vi "RegisterZeroWrite.vi"(7 "Data":T1 {"Data" max=127 format="%.0x"; "Slave Address" max=15 format="%.0x"}, 8 "error in (no error)":errorcluster, 9 "Number of Samples In":i32, 10 "Data Array":u8[][](array[numeric]), 11 "RFFE_Data In":T2 {"Toggle (high to low)" items=["0", "1", "Z", "L", "H", "X", "T", "V"]; "X Array" items=["0", "1", "Z", "L", "H", "X", "T", "V"]; "Z Array" items=["0", "1", "Z", "L", "H", "X", "T", "V"]; "L Array" items=["0", "1", "Z", "L", "H", "X", "T", "V"]; "H Array" items=["0", "1", "Z", "L", "H", "X", "T", "V"]; "One Array" items=["0", "1", "Z", "L", "H", "X", "T", "V"]; "Zero Array" items=["0", "1", "Z", "L", "H", "X", "T", "V"]}) -> (0 "error out":errorcluster, 1 "Number of Samples Out":i32, 2 "Data Array Out":u8[][](array[numeric]), 3 "RFFE_Data Out":T2 {"Toggle (high to low)" items=["0", "1", "Z", "L", "H", "X", "T", "V"]; "X Array" items=["0", "1", "Z", "L", "H", "X", "T", "V"]; "Z Array" items=["0", "1", "Z", "L", "H", "X", "T", "V"]; "L Array" items=["0", "1", "Z", "L", "H", "X", "T", "V"]; "H Array" items=["0", "1", "Z", "L", "H", "X", "T", "V"]; "One Array" items=["0", "1", "Z", "L", "H", "X", "T", "V"]; "Zero Array" items=["0", "1", "Z", "L", "H", "X", "T", "V"]})   [LabVIEW 2011]
doc: "Builds MIPI RFFE Register 0 Write with the specified data."
uses:
  Ctrls/RFFE_Data.ctl
  Ctrls/ClockDataChannels.ctl
  Ctrls/RegZeroWrite.ctl
  Ctrls/Commands.ctl
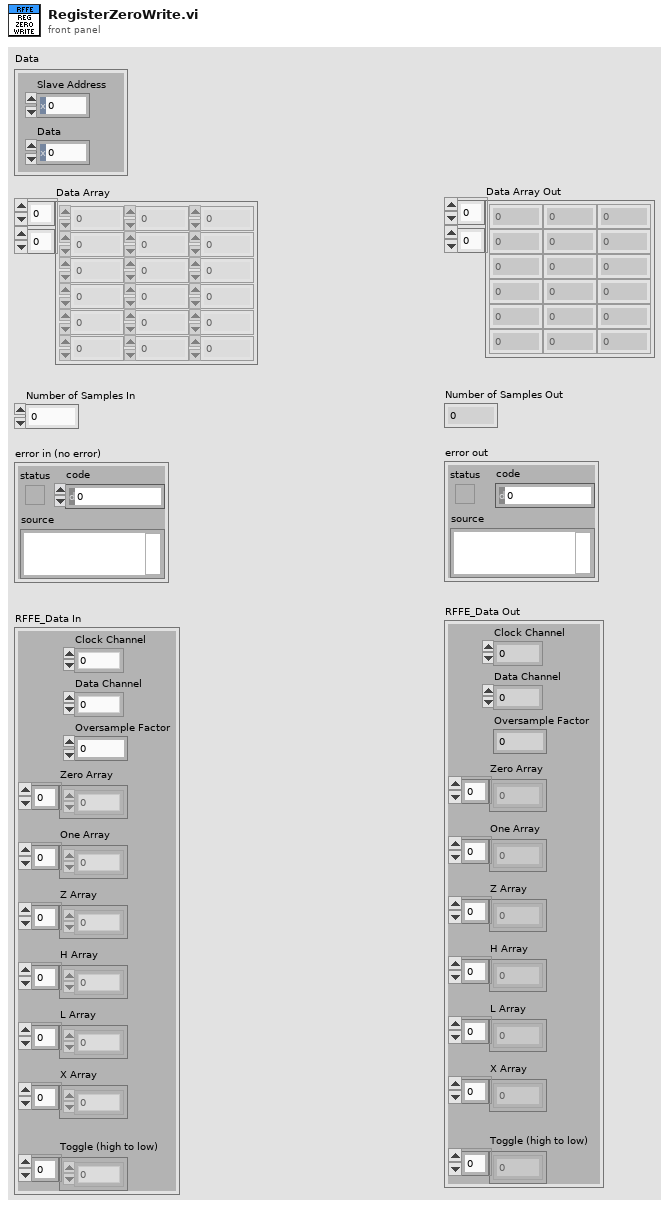
[diagram p1: front panel]
types:
  T1 = typedef "RegZeroWrite.ctl" = cluster{"Slave Address":u8, "Data":u8}
  T2 = typedef "RFFE_Data.ctl" = cluster{"Clock Channel":T3, "Data Channel":T3, "Oversample Factor":u8, "Zero Array":u8[], "One Array":u8[], "Z Array ":u8[], "H Array":u8[], "L Array":u8[], "X Array":u8[], "Toggle (high to low)":u8[]}
  T3 = typedef "ClockDataChannels.ctl" = enum16{"0", "1"}
  T4 = typedef "Commands.ctl" = cluster{"Command":enum16{"Extended Register Write", "Extended Register Read", "Extended Register Write Long", "Extended Register Read Long", "Register Write", "Register Read", "Register 0 Write"}, "Data/Address/ByteCount":u8}
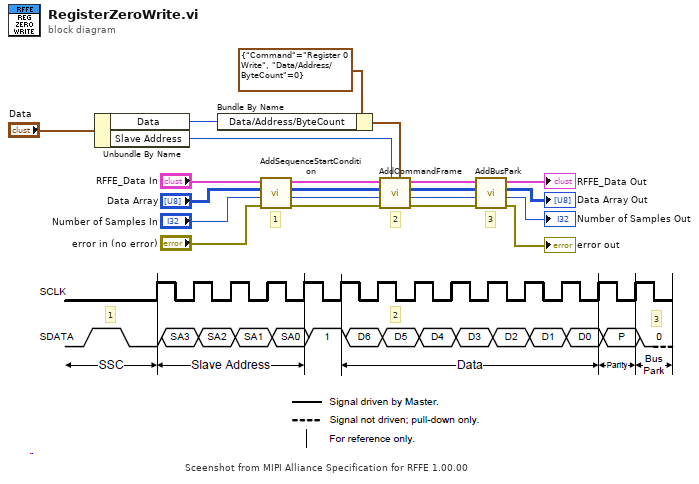
[diagram p0: block diagram]
diagram:
  # "1"
  # "3"
  # "2"
  # "Sceenshot from MIPI Alliance Specification for RFFE 1.00.00"
  # "3"
  # "2"
  # "1"
  n1 = Unbundle By Name("Data") -> ("Data"=w12:u8, "Slave Address"=w1:u8)
  n2 = Bundle By Name(cluster=T4 {"Command"=enum."Register 0 Write", "Data/Address/ByteCount"=0} ("Command"), "Data/Address/ByteCount"=w12) -> (w2:T4)
  n3 = call "AddSequenceStartCondition.vi"("error in (no error)"="error in (no error)", "Number of Samples In"="Number of Samples In", "Data Array In"="Data Array", "RFFE_Data In"="RFFE_Data In") -> ("error out"=w16:errorcluster, "Number of Samples Out"=w19:i32, "Data Array Out"=w17:u8[][], "RFFE_Data Out"=w18:T2)  [unwired: 4 in]
  n4 = call "AddCommandFrame.vi"("Command"=w2, "Slave Address"=w1, "error in (no error)"=w16, "Number of Samples In"=w19, "Data Array In"=w17, "RFFE_Data"=w18) -> ("error out"=w6:errorcluster, "Number of Samples Out"=w4:i32, "Data Array Out"=w5:u8[][], "Configuratation Out"=w7:T2)  [unwired: 2 in]
  n5 = call "AddBusPark.vi"("error in (no error)"=w6, "Number of Samples In"=w4, "Data Array In"=w5, "RFFE_Data In"=w7) -> ("error out"=→"error out":errorcluster, "Number of Samples Out"=→"Number of Samples Out":i32, "Data Array Out"=→"Data Array Out":u8[][], "RFFE_Data Out"=→"RFFE_Data Out":T2)  [unwired: 4 in]
